vi "Extract GPIB Address.VI"(8 "error in (no error)":errorcluster, 11 "VISA resource name":refnum<visa-resource-name>) -> (0 "error out":errorcluster, 1 "GPIB Board":u16, 2 "GPIB address":u16, 3 "VISA resource name out":refnum<visa-resource-name>)   [LabVIEW 2018, in "Agilent 87XX Series.lvlib"]
uses:
  Agilent 87XX Series.lvlib
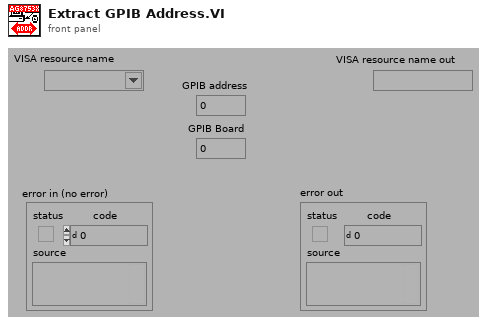
[diagram p1: front panel]
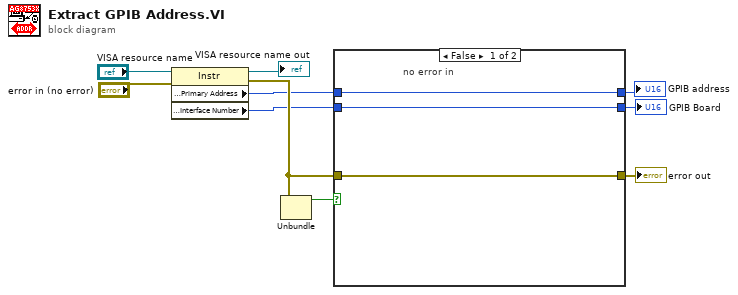
[diagram p0: block diagram]
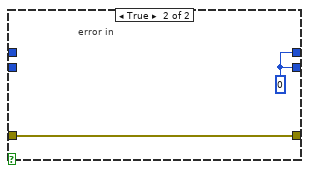
[diagram p2: hidden frame]
diagram:
  n1 = property class="Instr"(reference="VISA resource name", error in="error in (no error)") -> (reference out=→"VISA resource name out":refnum<visa-resource-name>, error out=w3:errorcluster, "GPIB Settings:Primary Address"=w2:u16, "Interface Information:Interface Number"=w1:u16)
  n2 = Unbundle(w3) -> ("status"=w10:bool)  [unwired: 2 out]
  n3 = case shown="False" w10 {
    tunnel: [w12 w14] -> w8
    tunnel: w3 -> [w13 w15]
    tunnel: [w13 w15] -> w9
    tunnel: [w11 w14] -> w7
    tunnel: w2 -> [w12 _]
    tunnel: w1 -> [w11 _]
    frame False {
      # "no error in"
    }
    frame True {
      w14 = u16 0
      # "error in"
    }
  }
  "error out" <- w9
  "GPIB address" <- w8
  "GPIB Board" <- w7
